vi "DAC_Xmit_orders.vi"(2 "Orders in":u64[](array[numeric]), 3 "FPGA VI Reference In":T1) -> (0 "error out":errorcluster, 1 "FPGA VI Reference Out":T1)   [LabVIEW 2013]
uses:
  fpga-bitfile-ref.ctl
  <vilib>/rvi/interface/common/niFpgaWaitOnOcc.vi
  <vilib>/Utility/error.llb/Error Cluster From Error Code.vi
  <vilib>/rvi/errors/niLvFpgaAdjustHostInterfaceError.vi
  <vilib>/RVI Host/nirviSupport.llb/nirviErrorClusterFromErrorCode.vi
  <vilib>/rvi/interface/nirviMethod/nirviMethod.xnode
  FPGA Bitfiles/FPGA_new_main_sbRIO_9612_10MHz_6us.lvbitx
  <vilib>/rvi/interface/nirviMethod/StockFPGA_InlinedMethodWaitForSingleIRQ.vi
  <vilib>/FPGAPlugInAG/sbRIO-9612/niLvFpga_WaitOnIrq_sbRIO-9612.vi
  <vilib>/FPGAPlugInAG/sbRIO-9612/niLvFpga_AcknowledgeIrq_sbRIO-9612.vi
  <vilib>/FPGAPlugInAG/sbRIO-9612/niLvFpga_WriteFifo_sbRIO-9612.vi
  <vilib>/rvi/errors/niLvFpgaMergeErrorWithErrorCode.vi
panel:
  in  "stop":bool
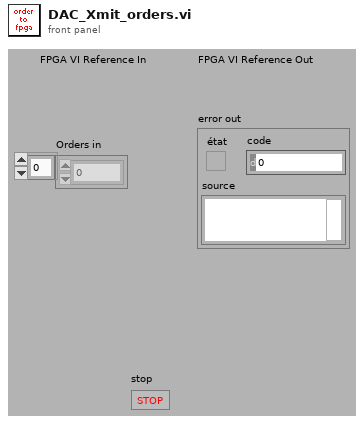
[diagram p1: front panel]
types:
  T1 = typedef "fpga-bitfile-ref.ctl" = refnum<k20>
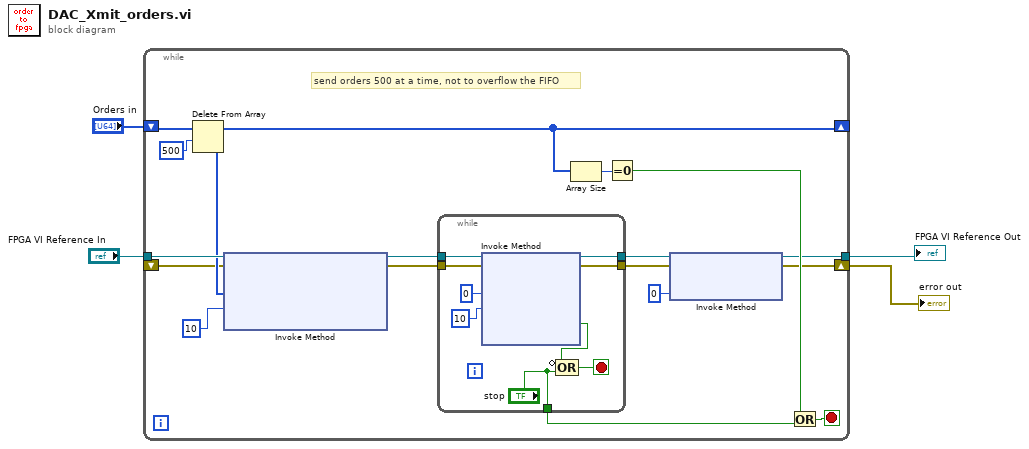
[diagram p0: block diagram]
diagram:
  n1 = while {
    tunnel: "FPGA VI Reference In" -> [w20]
    tunnel: [w8] -> w3
    shift-right: [w15] -> _
    shift-left: "Orders in" -> [w18]
    shift-right: [w7] -> w2
    shift-left: _ -> [w5]
    stop <- w12 stop-if-true
    # "send orders 500 at a time, not to overflow the FIFO"
    n2 = Delete From Array(array=w18, length=500) -> (deleted portion=w16:u64[], array with subset deleted=w15:u64[])  [unwired: 1 in]
    n3 = xnode "Invoke Method"("FPGA VI Reference In"=w20, "error in"=w5, "Data"=w16, "Timeout (ms)"=10) -> ("FPGA VI Reference Out"=w22:T1, "error out"=w21:errorcluster)  [unwired: 1 out]
    n4 = while {
      tunnel: w22 -> [w31]
      tunnel: [w30] -> w10
      tunnel: [w29] -> w9
      tunnel: w21 -> [w28]
      tunnel: ["stop"] -> w13
      stop <- w25 stop-if-true
      n5 = xnode "Invoke Method"("FPGA VI Reference In"=w31, "error in"=w28, "IRQ Number(s)"=0, "Timeout (ms)"=10) -> ("FPGA VI Reference Out"=w30:T1, "error out"=w29:errorcluster, "Timed Out"=w24:bool)  [unwired: 1 out]
      n6 = Compound Arithmetic op=OR(invert w24, "stop") -> (w25:bool)
    }
    n7 = Array Size(array=w15) -> (size(s)=w14:i32)
    n8 = Equal To 0?(x=w14) -> (x = 0?=w11:bool)
    n9 = xnode "Invoke Method"("FPGA VI Reference In"=w10, "error in"=w9, "IRQ Number(s)"=0) -> ("FPGA VI Reference Out"=w8:T1, "error out"=w7:errorcluster)
    n10 = Or(x=w11, y=w13) -> (x .or. y?=w12:bool)
  }
  "error out" <- w2
  "FPGA VI Reference Out" <- w3
